vi "InitialSetup.vi"   [LabVIEW 2015]
uses:
  <userlib>/Newport ESP301/Newport ESP301.lvlib
panel:
  # "You dont have to run this if you haven't taken the camera out or bumped things.\nYou do have to run this if you did not run the DailyEnd program before turning the box off last time."
  # "Run this before you align and set up the camera and lens with the callibration slide."
  # "With the ESP301 on, run this program and it will find and set the mid point of all axes to zero."
types:
  T1 = enum16{"Find +0 Position Count", "Find Home and Index Signals", "Find Home Signal", "Find Positive Limit Signal", "Find Negative Limit Signal", "Find Positve Limit and Index Signals", "Find Negative Limit and Index Signals"}
  T2 = enum16{"Trapezoidal Mode", "S-curve Mode", "Jog Mode", "Slave to master's desired position (trajectory)", "Slave to master's actual position (feedback)", "Slave to master's actual velocity for jogging"}
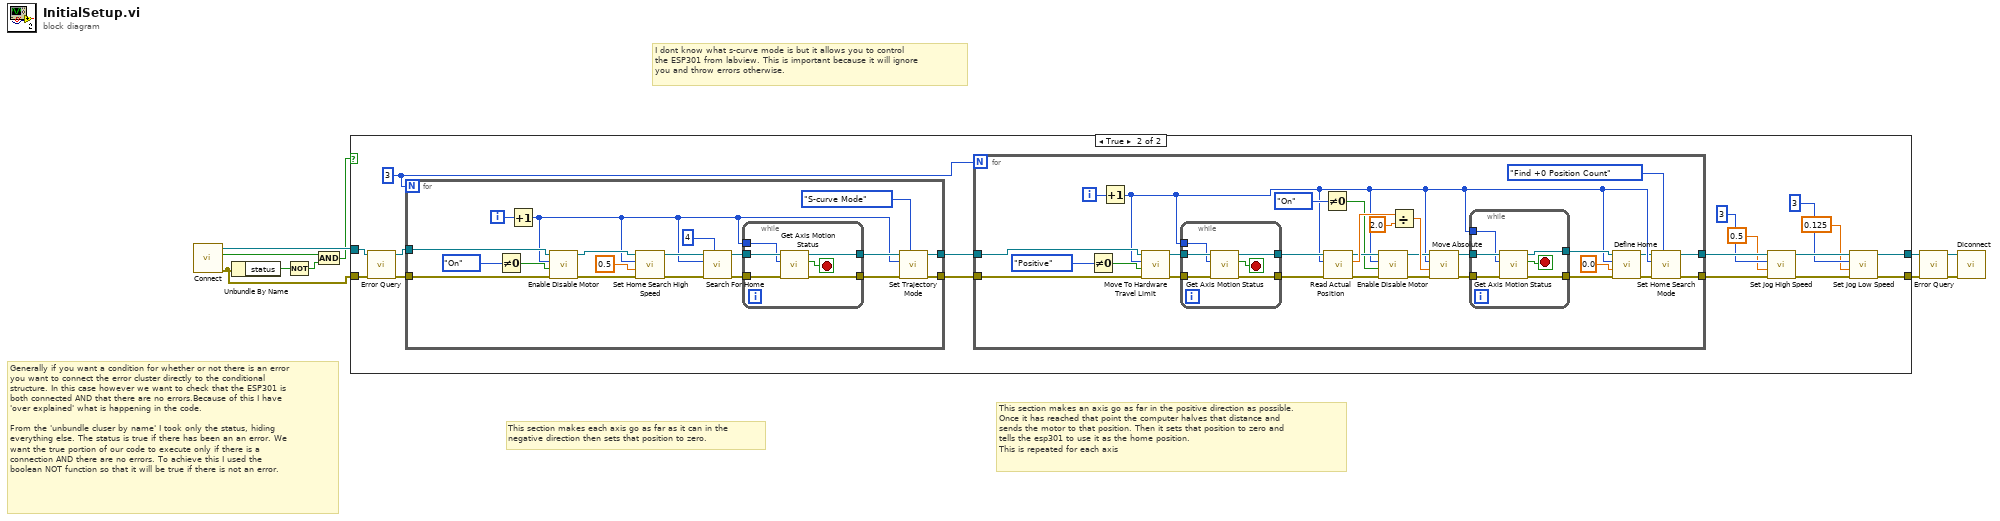
[diagram p0: block diagram]
diagram:
  # "This section makes an axis go as far in the positive direction as possible. \nOnce it has reached that point the computer halves that distance and\nsends the motor to that position. Then it sets that position to zero and \ntells the esp301 to use it as the home position. \nThis is repeated for each axis"
  # "This section makes each axis go as far as it can in the \nnegative direction then sets that position to zero."
  # "I dont know what s-curve mode is but it allows you to control \nthe ESP301 from labview. This is important because it will ignore \nyou and throw errors otherwise."
  # "Generally if you want a condition for whether or not there is an error\nyou want to connect the error cluster directly to the conditional\nstructure. In this case however we want to check that the ESP301 is\nboth connected AND that there are no errors.Because of this I have\n'over explained' what is happening in the code.\n\nFrom the 'unbundle cluser by name' I took only the status, hiding \neverything else. The status is true if there has been an an error. We\nwant the true portion of our code to execute only if there is a \nconnection AND there are no errors. To achieve this I used the \nboolean NOT function so that it will be true if there is not an error."
  n1 = call "Connect.vi"() -> ("error out"=w9:errorcluster, "Connected"=w1:bool, "VISA resource name out"=w10:refnum<visa-resource-name>)  [unwired: 5 in]
  n2 = Unbundle By Name(w9) -> ("status"=w8:bool)
  n3 = Not(x=w8) -> (.not. x?=w2:bool)
  n4 = And(x=w1, y=w2) -> (x .and. y?=w3:bool)
  n5 = case shown="True" w3 {
    tunnel: w10 -> [w12 w13]
    tunnel: w9 -> [w11 w16]
    tunnel: [w12 w21] -> w7
    tunnel: [w11 w22] -> w6
    frame False {
    }
    frame True {
      w29 = 3
      n6 = call <userlib>:"Error Query.vi"("error in (no error)"=w16, "VISA resource name"=w13) -> ("error out"=w15:errorcluster, "VISA resource name out"=w14:refnum<visa-resource-name>)  [unwired: 2 in, 2 out]
      n7 = for {
        N: w29 -> [_]
        tunnel: w14 -> [w78]
        tunnel: w15 -> [w77]
        tunnel: [w84] -> w28
        tunnel: [w83] -> w27
        i -> [w89]
        n8 = Not Equal To 0?(x=enum16{"Off", "On"}."On") -> (x != 0?=w72:bool)
        n9 = Increment(x=w89) -> (x+1=w74:i32)
        n10 = call <userlib>:"Enable Disable Motor.vi"("error in (no error)"=w77, "Action (F - OFF)"=w72, "Axis (1)"=w74, "VISA resource name"=w78) -> ("error out"=w75:errorcluster, "VISA resource name out"=w76:refnum<visa-resource-name>)  [unwired: 2 in]
        n11 = call <userlib>:"Set Home Search High Speed.vi"("error in (no error)"=w75, "Search High Speed (0 units/s)"=0.5, "Axis (1)"=w74, "VISA resource name"=w76) -> ("error out"=w87:errorcluster, "VISA resource name out"=w88:refnum<visa-resource-name>)  [unwired: 2 in]
        n12 = call <userlib>:"Search For Home.vi"("Home mode"=4, "error in (no error)"=w87, "Axis (1)"=w74, "VISA resource name"=w88) -> ("error out"=w81:errorcluster, "VISA resource name out"=w82:refnum<visa-resource-name>)  [unwired: 3 in]
        n13 = while {
          tunnel: w82 -> [w95]
          tunnel: w81 -> [w94]
          tunnel: w74 -> [w93]
          tunnel: [w92] -> w80
          tunnel: [w91] -> w79
          stop <- w90 stop-if-true
          n14 = call <userlib>:"Get Axis Motion Status.vi"("error in (no error)"=w94, "Axis (1)"=w93, "VISA resource name"=w95) -> ("error out"=w91:errorcluster, "Motion Done"=w90:bool, "VISA resource name out"=w92:refnum<visa-resource-name>)  [unwired: 2 in]
        }
        n15 = call <userlib>:"Set Trajectory Mode.vi"("Trajectory Mode"=T2."S-curve Mode", "error in (no error)"=w79, "Axis (1)"=w74, "VISA resource name"=w80) -> ("error out"=w83:errorcluster, "VISA resource name out"=w84:refnum<visa-resource-name>)  [unwired: 3 in]
      }
      n16 = for {
        N: w29 -> [_]
        tunnel: w28 -> [w57]
        tunnel: w27 -> [w56]
        tunnel: [w32] -> w25
        tunnel: [w31] -> w26
        i -> [w58]
        n17 = Not Equal To 0?(x=enum16{"Negative", "Positive"}."Positive") -> (x != 0?=w36:bool)
        n18 = Increment(x=w58) -> (x+1=w35:i32)
        n19 = call <userlib>:"Move To Hardware Travel Limit.vi"("error in (no error)"=w56, "Move Direction (+)"=w36, "Axis (1)"=w35, "VISA resource name"=w57) -> ("error out"=w54:errorcluster, "VISA resource name out"=w55:refnum<visa-resource-name>)  [unwired: 2 in]
        n20 = while {
          tunnel: w55 -> [w70]
          tunnel: w54 -> [w69]
          tunnel: w35 -> [w68]
          tunnel: [w67] -> w53
          tunnel: [w66] -> w52
          stop <- w65 stop-if-true
          n21 = call <userlib>:"Get Axis Motion Status.vi"("error in (no error)"=w69, "Axis (1)"=w68, "VISA resource name"=w70) -> ("error out"=w66:errorcluster, "Motion Done"=w65:bool, "VISA resource name out"=w67:refnum<visa-resource-name>)  [unwired: 2 in]
        }
        n22 = Not Equal To 0?(x=enum16{"Off", "On"}."On") -> (x != 0?=w38:bool)
        n23 = call <userlib>:"Read Actual Position.vi"("error in (no error)"=w52, "Axis (1)"=w35, "VISA resource name"=w53) -> ("error out"=w45:errorcluster, "Position (units)"=w51:dbl, "VISA resource name out"=w46:refnum<visa-resource-name>)  [unwired: 2 in]
        n24 = call <userlib>:"Enable Disable Motor.vi"("error in (no error)"=w45, "Action (F - OFF)"=w38, "Axis (1)"=w35, "VISA resource name"=w46) -> ("error out"=w44:errorcluster, "VISA resource name out"=w43:refnum<visa-resource-name>)  [unwired: 2 in]
        n25 = Divide(x=w51, y=2.0) -> (x/y=w49:dbl)
        n26 = call <userlib>:"Move Absolute.vi"("error in (no error)"=w44, "Position (0 units)"=w49, "Axis (1)"=w35, "VISA resource name"=w43) -> ("error out"=w47:errorcluster, "VISA resource name out"=w48:refnum<visa-resource-name>)  [unwired: 2 in]
        n27 = while {
          tunnel: w48 -> [w64]
          tunnel: w47 -> [w63]
          tunnel: w35 -> [w62]
          tunnel: [w61] -> w42
          tunnel: [w60] -> w41
          stop <- w59 stop-if-true
          n28 = call <userlib>:"Get Axis Motion Status.vi"("error in (no error)"=w63, "Axis (1)"=w62, "VISA resource name"=w64) -> ("error out"=w60:errorcluster, "Motion Done"=w59:bool, "VISA resource name out"=w61:refnum<visa-resource-name>)  [unwired: 2 in]
        }
        n29 = call <userlib>:"Define Home.vi"("error in (no error)"=w41, "Home Position (0 units)"=0.0, "Axis (1)"=w35, "VISA resource name"=w42) -> ("error out"=w33:errorcluster, "VISA resource name out"=w34:refnum<visa-resource-name>)  [unwired: 2 in]
        n30 = call <userlib>:"Set Home Search Mode.vi"("Home mode"=T1."Find +0 Position Count", "error in (no error)"=w33, "Axis (1)"=w35, "VISA resource name"=w34) -> ("error out"=w31:errorcluster, "VISA resource name out"=w32:refnum<visa-resource-name>)  [unwired: 3 in]
      }
      n31 = call <userlib>:"Set Jog High Speed.vi"("error in (no error)"=w26, "Jog High Speed (0 units/s)"=0.5, "Axis (1)"=3, "VISA resource name"=w25) -> ("error out"=w19:errorcluster, "VISA resource name out"=w20:refnum<visa-resource-name>)  [unwired: 2 in]
      n32 = call <userlib>:"Set Jog Low Speed.vi"("error in (no error)"=w19, "Jog Low Speed (0 units/s)"=0.125, "Axis (1)"=3, "VISA resource name"=w20) -> ("error out"=w22:errorcluster, "VISA resource name out"=w21:refnum<visa-resource-name>)  [unwired: 2 in]
    }
  }
  n33 = call <userlib>:"Error Query.vi"("error in (no error)"=w6, "VISA resource name"=w7) -> ("error out"=w5:errorcluster, "VISA resource name out"=w4:refnum<visa-resource-name>)  [unwired: 2 in, 2 out]
  n34 = call "Diconnect.vi"("error in (no error)"=w5, "VISA resource name"=w4) -> ()  [unwired: 6 in]
